vi "initialize Session Data.vi"(0 "Session in":refnum<class "Engine.lvclass">, 11 "error in":errorcluster) -> (4 "Session out":refnum<class "Engine.lvclass">, 15 "error out":errorcluster)   [LabVIEW 2020, in "TSS.lvlib" / "Engine.lvclass"]
uses:
  Engine.lvclass
  Execution/Typedefs/Session Handle.ctl
  Execution/Execution.lvclass
  Engine.lvclass/Engine.ctl
  <userlib>/_Session Fwk/Session - Root.lvclass
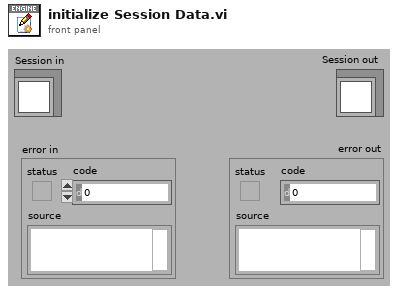
[diagram p1: front panel]
types:
  T1 = typedef "TSS.lvlib/Execution.lvclass/Session Handle.ctl" = refnum<data-value>
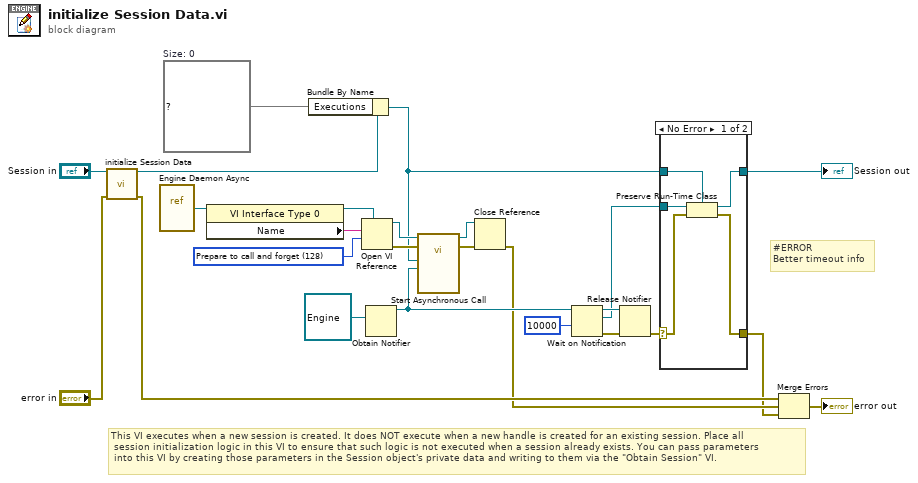
[diagram p0: block diagram]
diagram:
  w1 = set{T1} {}  # Size: 0
  w17 = 128 items=["Record modifications"=1, "Open templates for editing"=2, "Prompt user to save"=4, "Prepare for reentrant run"=8, "Prompt to find missing subVIs"=16, "Hide loading dialog box"=32, "Enable simultaneous calls"=64, "Prepare to call and forget"=128, "Simultaneous call and forget"=192, "Prepare to call and collect"=256, "Simultaneous call and collect"=320]
  # "#ERROR\nBetter timeout info"
  # "This VI executes when a new session is created. It does NOT execute when a new handle is created for an existing session. Place all\n session initialization logic in this VI to ensure that such logic is not executed when a session already exists. You can pass parameters\n into this VI by creating those parameters in the Session object's private data and writing to them via the \"Obtain Session\" VI."
  n1 = call-parent "initialize Session Data.vi"("OBJ - Session in"="Session in", "error in"="error in") -> ("OBJ - Session out"=w3:refnum<class "Engine.lvclass">, "error out"=w25:errorcluster)  [unwired: 12 in]
  n2 = vi-ref "Engine Daemon Async.vi"() -> (w15:refnum<vi>)
  n3 = property class="VI Interface Type 0"(reference=w15) -> (reference out=w18:refnum<vi>, "Name"=w16:string)  [unwired: 1 in, 1 out]
  n4 = Bundle By Name(cluster=w3, "Executions"=w1) -> (w2:refnum<class "Engine.lvclass">)
  n5 = Open VI Reference(type specifier VI Refnum (for type only)=w18, vi path=w16, options=w17) -> (vi reference=w20:refnum<vi>, error out=w19:errorcluster)  [unwired: 3 in]
  n6 = Obtain Notifier(notification data type=refnum<class "Engine.lvclass"> refnum ("TSEngine")) -> (notifier out=w9:refnum<notifier>)  [unwired: 3 in, 2 out]
  n7 = call-by-ref "Start Asynchronous Call"(reference=w20, error in=w19, "Daemon Notifier"=w9, "TSEngine in"=w2) -> (reference out=w22:refnum<vi>, error out=w21:errorcluster)  [unwired: 10 in]
  n8 = Close Reference(reference=w22, error in (no error)=w21) -> (error out=w8:errorcluster)
  n9 = Wait on Notification(notifier=w9, timeout in ms (-1)=10000) -> (notifier out=w14:refnum<notifier>, notification=w6:refnum<class "Engine.lvclass">, error out=w13:errorcluster)  [unwired: 2 in, 1 out]
  n10 = Release Notifier(notifier=w14, error in (no error)=w13) -> (error out=w7:errorcluster)  [unwired: 1 in, 2 out]
  n11 = case shown="No Error" w7 {
    selector: w7 -> [w27 w31]
    tunnel: w6 -> [w30 _]
    tunnel: w2 -> [w29 w32]
    tunnel: [w28 w32] -> w5
    tunnel: [w26 w31] -> w4
    frame No Error {
      n12 = Preserve Run-Time Class(object in=w30, error in=w27, 2:w29) -> (object out=w28:refnum<class "Engine.lvclass">, error out=w26:errorcluster)
    }
    frame Error {
    }
  }
  "Session out" <- w5
  n13 = Merge Errors(w25, w8, w4) -> (→"error out":errorcluster)
